vi "FpsMeas.vi"() -> (1 "FPS":dbl)   [LabVIEW 2024]
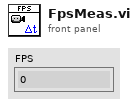
[diagram p1: front panel]
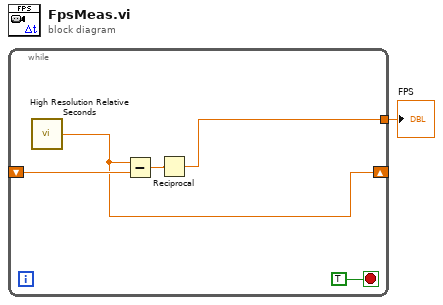
[diagram p0: block diagram]
diagram:
  n1 = while {
    shift-right: [w2] -> _
    shift-left: _ -> [w4]
    tunnel: [w3] -> w1
    stop <- TRUE stop-if-true
    n2 = call <vilib>:"High Resolution Relative Seconds.vi"() -> ("relative seconds"=w2:dbl)
    n3 = Subtract(x=w2, y=w4) -> (x-y=w5:dbl)
    n4 = Reciprocal(x=w5) -> (1/x=w3:dbl)
  }
  "FPS" <- w1
